vi "1 Tap 48-Bit RGB.vi"() -> ()   [LabVIEW 2014]
uses:
  <vilib>/rvi/eio/common/nirviEmuTemplateMethod_errors.vi
  <vilib>/eio/EIONode/EIONode.xnode
panel:
  out "PixelData":u64
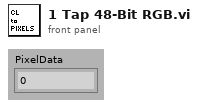
[diagram p1: front panel]
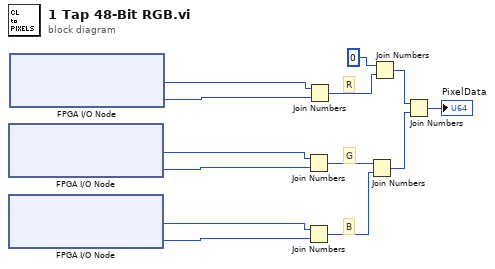
[diagram p0: block diagram]
diagram:
  # "B"
  # "R"
  # "G"
  n1 = xnode "FPGA I/O Node"() -> ("IO Module\\CL Port E"=w2:u8, "IO Module\\CL Port D"=w6:u8)  [unwired: 2 in, 2 out]
  n2 = xnode "FPGA I/O Node"() -> ("IO Module\\CL Port F"=w1:u8, "IO Module\\CL Port C"=w5:u8)  [unwired: 2 in, 2 out]
  n3 = xnode "FPGA I/O Node"() -> ("IO Module\\CL Port B"=w3:u8, "IO Module\\CL Port A"=w13:u8)  [unwired: 2 in, 2 out]
  n4 = Join Numbers(hi=w2, lo=w6) -> ((hi.lo)=w11:u16)
  n5 = Join Numbers(hi=w1, lo=w5) -> ((hi.lo)=w4:u16)
  n6 = Join Numbers(hi=w3, lo=w13) -> ((hi.lo)=w12:u16)
  n7 = Join Numbers(hi=w11, lo=w4) -> ((hi.lo)=w7:u32)
  n8 = Join Numbers(hi=u16 0, lo=w12) -> ((hi.lo)=w9:u32)
  n9 = Join Numbers(hi=w9, lo=w7) -> ((hi.lo)=→"PixelData":u64)
